vi "main_grid_forming_PQ_bu.vi"() -> ()   [LabVIEW 2021]
uses:
  <vilib>/xnet/xnet.llb/XNET Frame CAN.ctl
  <vilib>/xnet/xnet.llb/XNET Frame Type CAN.ctl
  Helper functions/General Purpose/references.ctl
  Helper functions/General Purpose/measurements.ctl
  Helper functions/Time-sync/time_sync/TypeDef/Synch_shift--cluster.ctl
  <vilib>/Platform/TimedLoop/XDataNode/timing_clust.ctl
  <vilib>/Platform/TimedLoop/XDataNode/nitl_modes.ctl
  <vilib>/Platform/TimedLoop/XDataNode/wakeup.ctl
  Helper functions/communication/AFE_froming_Central.ctl
  Helper functions/communication/AFE_froming_Central_Info.ctl
  Helper functions/communication/AFE_froming_Central_Data.ctl
  <vilib>/xnet/xnet.llb/XNET Write (Frame CAN).vi
  <vilib>/xnet/xnet.llb/XNET Read (Frame CAN).vi
  <vilib>/Platform/TimedLoop/XDataNode/XDataNode.xnode
  <vilib>/Platform/TimedLoop/XDataNode/XDNodeRunTimeDep.lvlib
  <userlib>/_OpenG.lib/boolean/boolean.llb/openg_boolean__ogtk.lvlib
panel:
  in  "Q2 bias":dbl=-800.0
  in  "delta V":dbl format="%#_13g"
  in  "delta f":dbl=0.005800000000000027 format="%#_13g"
  in  "biasQ4":dbl=200.0
  in  "biasV4":dbl
  in  "biasV1":dbl=0.6
  out "form":timestamp
  out "follow":timestamp
  out "time_afe":timestamp
  out "start following 1 pre":bool
  out "t_rising":timestamp
  out "t_risingedge":dbl
  out "Synch Monitor":string[][](table)
  in  "Loop Time":u32=125
  out "Error out":errorcluster
  in  "Timeout [ms]":i32=3000
  out "Offset from TR (ns)":dbl
  out "Status Out":T1
  out "CAN OUT":T2[](array[typedef]) {"payload" format="%x"; "timestamp" format="%<%.7X\n%x>T"; "type" items=["CAN Data"=0, "CAN Remote"=1, "CAN Bus Error"=2, "CAN 2.0 Data"=8, "CAN FD Data"=16, "CAN FD+BRS Data"=24, "J1939 Data"=192, "Delay"=224, "Log Trigger"=225, "Start Trigger"=226]; "identifier" format="%x"}
  in  "freq 1":dbl=50.0
  in  "Vabs 1":dbl=230.0
  in  "Varg 1":dbl
  in  "Start following 1":bool
  out "Forming 2":bool
  out "Forming 1":bool
  in  "Start forming 1":bool
  out "current time":timestamp
  in  "measurements":T4
  in  "references":T5
  in  "To ACT CH 4":bool
  in  "To ACT CH 3":bool
  in  "To ACT CH 2":bool
  out "Error 4":bool
  out "Fault 4":bool
  out "Error 3":bool
  out "Fault 3":bool
  out "Error 2":bool
  out "Fault 2":bool
  out "State code 4":i32
  out "State code 3":i32
  out "State code 2":i32
  out "State code 1":i32
  out "Error 1":bool
  out "Fault 1":bool
  in  "To ACT CH 1":bool
  in  "main stop":bool
  in  "Vdc4":dbl=750.0
  in  "Qac4":dbl
  in  "Pac3":dbl=750.0
  in  "Qac3":dbl
  in  "Pac2":dbl
  in  "Qac2":dbl
  in  "Emergency 4":bool
  in  "To IN OP  4":bool
  in  "SEND sp 4":bool
  in  "Clear 4":bool
  in  "Shutdwn 4":bool
  in  "Emergency 3":bool
  in  "To IN OP  3":bool
  in  "SEND sp 3":bool
  in  "Clear 3":bool
  in  "Shutdwn 3":bool
  in  "Emergency 2":bool
  in  "To IN OP  2":bool
  in  "SEND sp 2":bool
  in  "Clear 2":bool
  in  "Shutdwn 2":bool
  out "V slider 22":dbl(slide) caption="V-i" max=-10.0 scale=650.0..780.0 scale format="%#_4g"
  out "V slider 21":dbl(slide) caption="V-i" max=-10.0 scale=650.0..780.0 scale format="%#_4g"
  out "V slider 20":dbl(slide) caption="V-i" max=-10.0 scale=650.0..780.0 scale format="%#_4g"
  out "kW":dbl caption="Numeric" format="%#.3g"
  out "?VkVAr":dbl caption="Numeric" format="%.3g"
  out "kW":dbl caption="Numeric" format="%#.3g"
  out "?VkVAr":dbl caption="Numeric" format="%.3g"
  out "kW":dbl caption="Numeric" format="%#.3g"
  out "?VkVAr":dbl caption="Numeric" format="%.3g"
  out "OFF 4":bool
  out "ON 4":bool
  out "Ready 4":bool
  out "OFF 3":bool
  out "ON 3":bool
  out "Ready 3":bool
  out "OFF 2":bool
  out "ON 2":bool
  out "Ready 2":bool
  out "error out":errorcluster
  out "?VkVAr":dbl caption="Numeric" format="%.3g"
  out "kW":dbl caption="Numeric" format="%#.3g"
  out "V slider 19":dbl(slide) caption="V-i" max=-10.0 scale=650.0..780.0 scale format="%#_4g"
  in  "Vdc1":dbl=750.0
  out "OFF 1":bool
  out "ON 1":bool
  out "Ready 1":bool
  out "CAN IN":T2 {"payload" format="%x"; "timestamp" format="%<%.7X\n%x>T"; "type" items=["CAN Data"=0, "CAN Remote"=1, "CAN Bus Error"=2, "CAN 2.0 Data"=8, "CAN FD Data"=16, "CAN FD+BRS Data"=24, "J1939 Data"=192, "Delay"=224, "Log Trigger"=225, "Start Trigger"=226]; "identifier" format="%x"}
  in  "Emergency 1":bool
  in  "Qac1":dbl
  in  "conv":T6
  in  "CAN [ms]":i64=1
  out "CAN with Conv":bool
  out "Measurements":bool
  in  "Shutdwn 1":bool
  in  "Clear 1":bool
  in  "SEND sp 1":bool
  in  "To IN OP 1":bool
  out "logging":bool
  # "Resource agents: AFE 1-4"
  # "package identifiers:\n1xx VSC1 \n2xx VSC2\n3xx VSC3\n4xx VSC4\n\nx0x send from agent to resource\nx02 Power setpoints\nx06 Measurements\nx9 status\n          = [state; error; alarm; OFF; Ready; ON]\n\n \n\nx1x send from resource to agent\nx10 Power measurements\nx11 Measurements\nx12 status\n          = [state; error; alarm; full; precharge; neg; 0; 0]"
  # "B18"
  # "B 22\nB19"
  # "VSC 4"
  # "B17"
  # "B21"
  # "VSC 3"
  # "B16"
  # "B20"
  # "Start-up - Shut down"
  # "VSC 2"
  # "B15"
  # "B19"
  # "Start-up - Shut down"
  # "VSC 1"
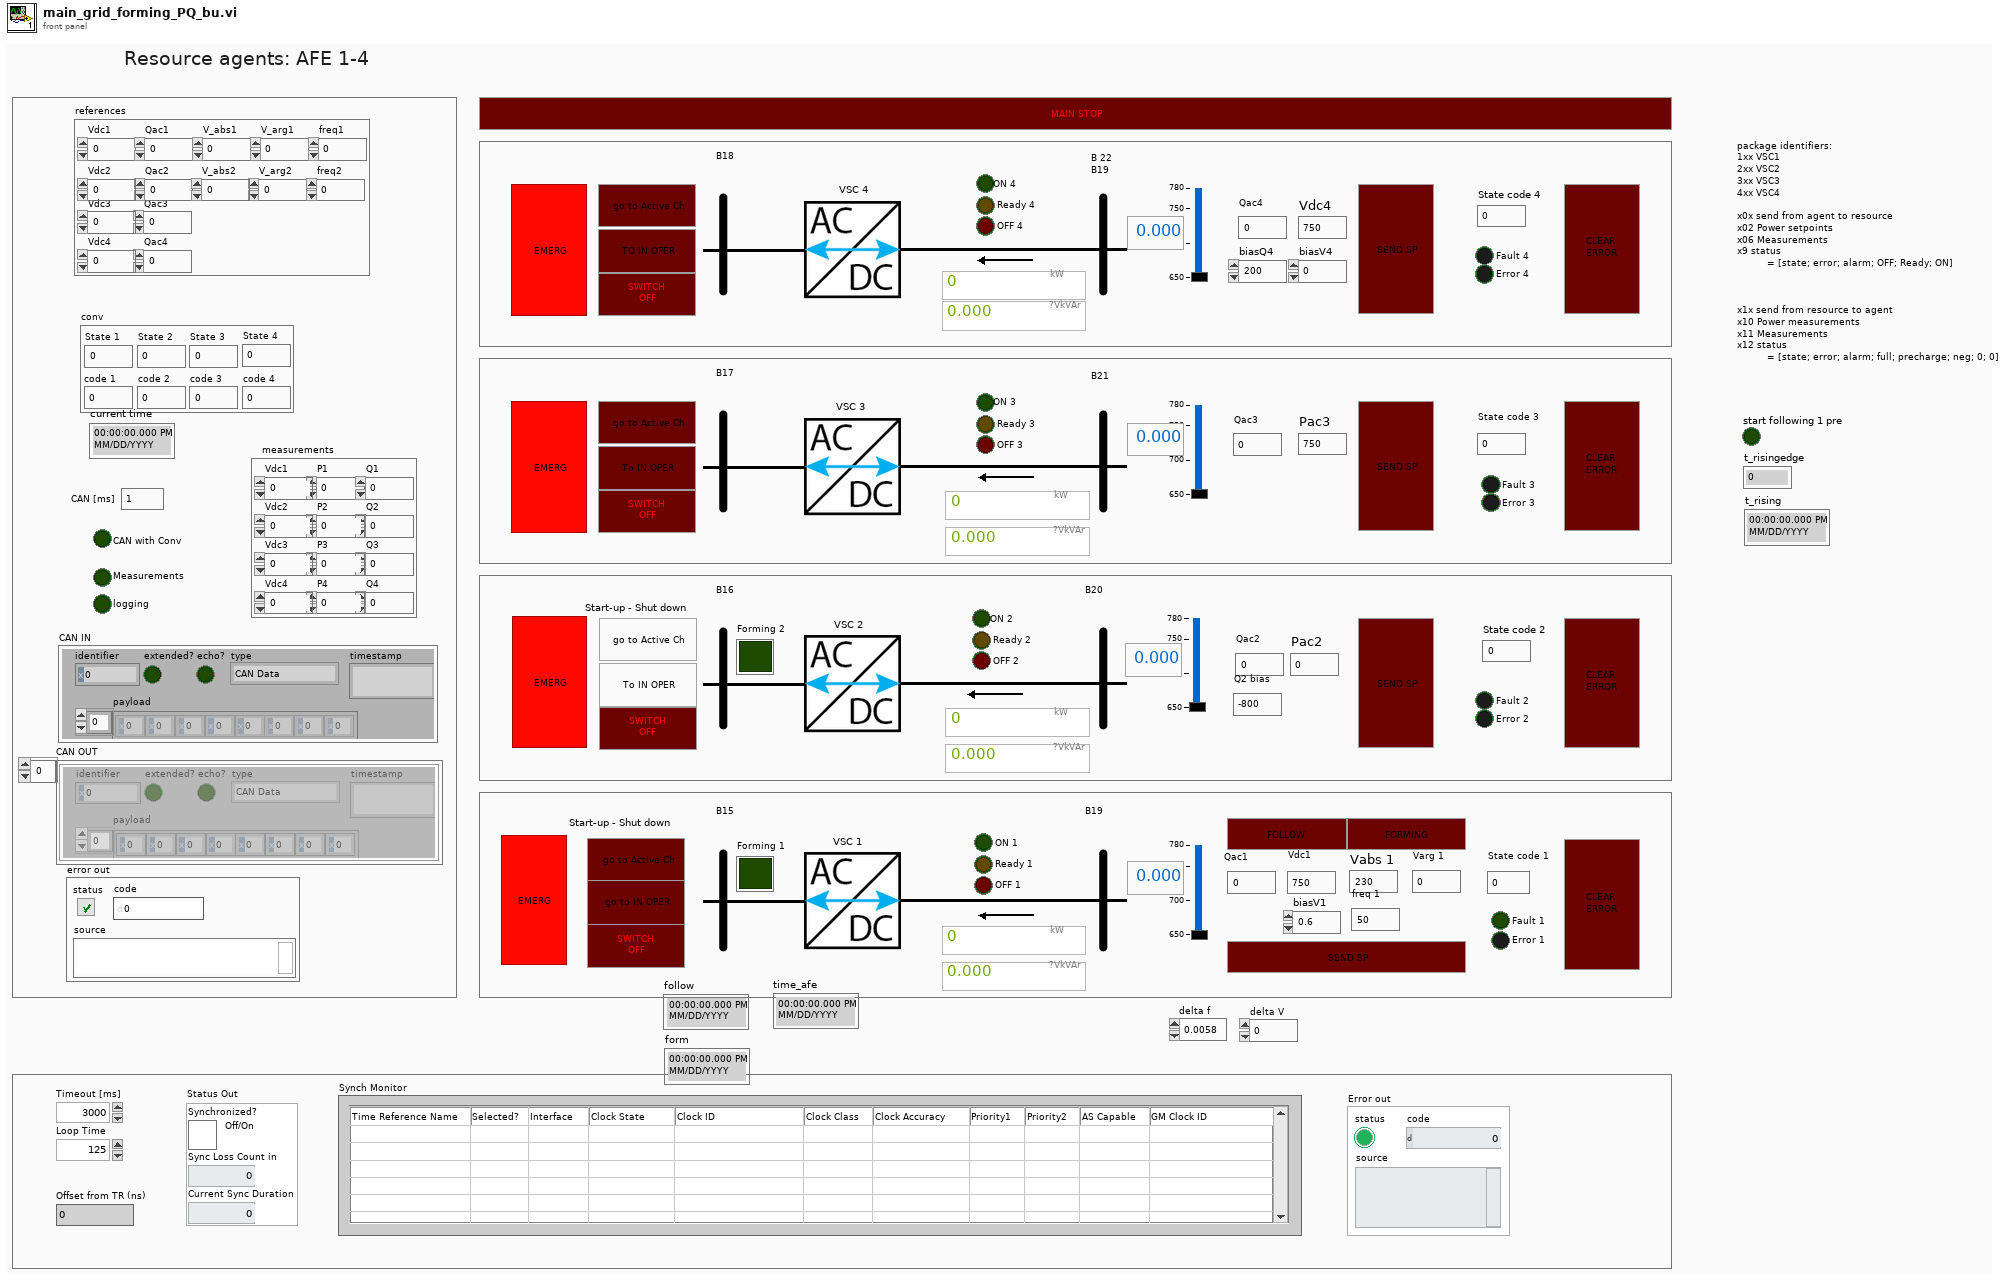
[diagram p1: front panel]
types:
  T1 = typedef "Synch_shift--cluster.ctl" = cluster{"Synchronized?":bool, "Sync Loss Count in":u32, "Current Sync Duration":u32}
  T2 = typedef "XNET Frame CAN.ctl" = cluster{"timestamp":timestamp, "payload":u8[], "identifier":u32, "type":T3, "extended?":bool, "echo?":bool}
  T3 = typedef "XNET Frame Type CAN.ctl" = u8
  T4 = typedef "measurements.ctl" = cluster{"Vdc1":dbl, "P1":dbl, "Vdc2":dbl, "P2":dbl, "Q2":dbl, "Vdc3":dbl, "P3":dbl, "Q3":dbl, "Vdc4":dbl, "P4":dbl, "Q4":dbl, "Q1":dbl}
  T5 = typedef "references.ctl" = cluster{"Vdc1":dbl, "Vdc2":dbl, "Qac2":dbl, "Vdc3":dbl, "Qac3":dbl, "Vdc4":dbl, "Qac4":dbl, "Qac1":dbl, "V_arg2":dbl, "V_abs2":dbl, "V_abs1":dbl, "V_arg1":dbl, "freq1":dbl, "freq2":dbl}
  T6 = cluster{"State 1":dbl, "code 1":dbl, "code 2":dbl, "code 3":dbl, "code 4":dbl, "State 2":dbl, "State 3":dbl, "State 4":dbl}
  T7 = cluster{"Frame In":refnum<k21>, "Frame Out":refnum<k21>}
  T8 = typedef "XDNodeRunTimeDep.lvlib/timing_clust.ctl" = cluster{"Expected End [f-1]":u64, "Actual End [f-1]":u64, "Finished Late? [f-1]":bool, "Expected End [i-1]":u64, "Actual End [i-1]":u64, "Finished Late? [i-1]":bool, "Expected Start [i]":u64, "Actual Start [i]":u64, "Expected Start [f]":u64, "Actual Start [f]":u64, "Source Name":string, "Structure Name":string, "Period":i64, "Deadline":i64, "Offset":i64, "Start":i64, "Priority":i32, "Timeout":i32, "Mode":T9, "Wakeup Reason":T10, "Error":errorcluster, "Source Type":string, "Secondary Source Type":string, "Global End Time":u64, "Global Start Time":u64, "Frame Duration":u64, "Iteration Duration":u64, "Assigned CPU":i32, "I/O Scan Engine Mode":u32}
  T9 = typedef "XDNodeRunTimeDep.lvlib/nitl_modes.ctl" = enum32{"No Change", "Process missed periods, maintain original phase", "Discard missed periods, maintain original phase", "Process missed periods, ignore original phase", "Discard missed periods, ignore original phase"}
  T10 = typedef "XDNodeRunTimeDep.lvlib/wakeup.ctl" = enum32{"Normal", "Aborted", "Asynchronous wakeup", "Timing source error", "Timed loop error", "Timeout"}
  T11 = typedef "AFE_froming_Central.ctl" = cluster{"Info":T12, "Data":T13}
  T12 = typedef "AFE_froming_Central_Info.ctl" = cluster{"Resource":string, "Problem":bool, "Timestamp":dbl}
  T13 = typedef "AFE_froming_Central_Data.ctl" = cluster{"Start forming 1":bool, "Forming/Following":bool[], "Start forming 2":bool, "measurements":cluster{"Vdc1":dbl, "P1":dbl, "Vdc2":dbl, "P2":dbl, "Q2":dbl, "Vdc3":dbl, "P3":dbl, "Q3":dbl, "Vdc4":dbl, "P4":dbl, "Q4":dbl, "Q1":dbl}, "Status":bool[], "references":T5, "Start following 1":bool, "Start following 2":bool}
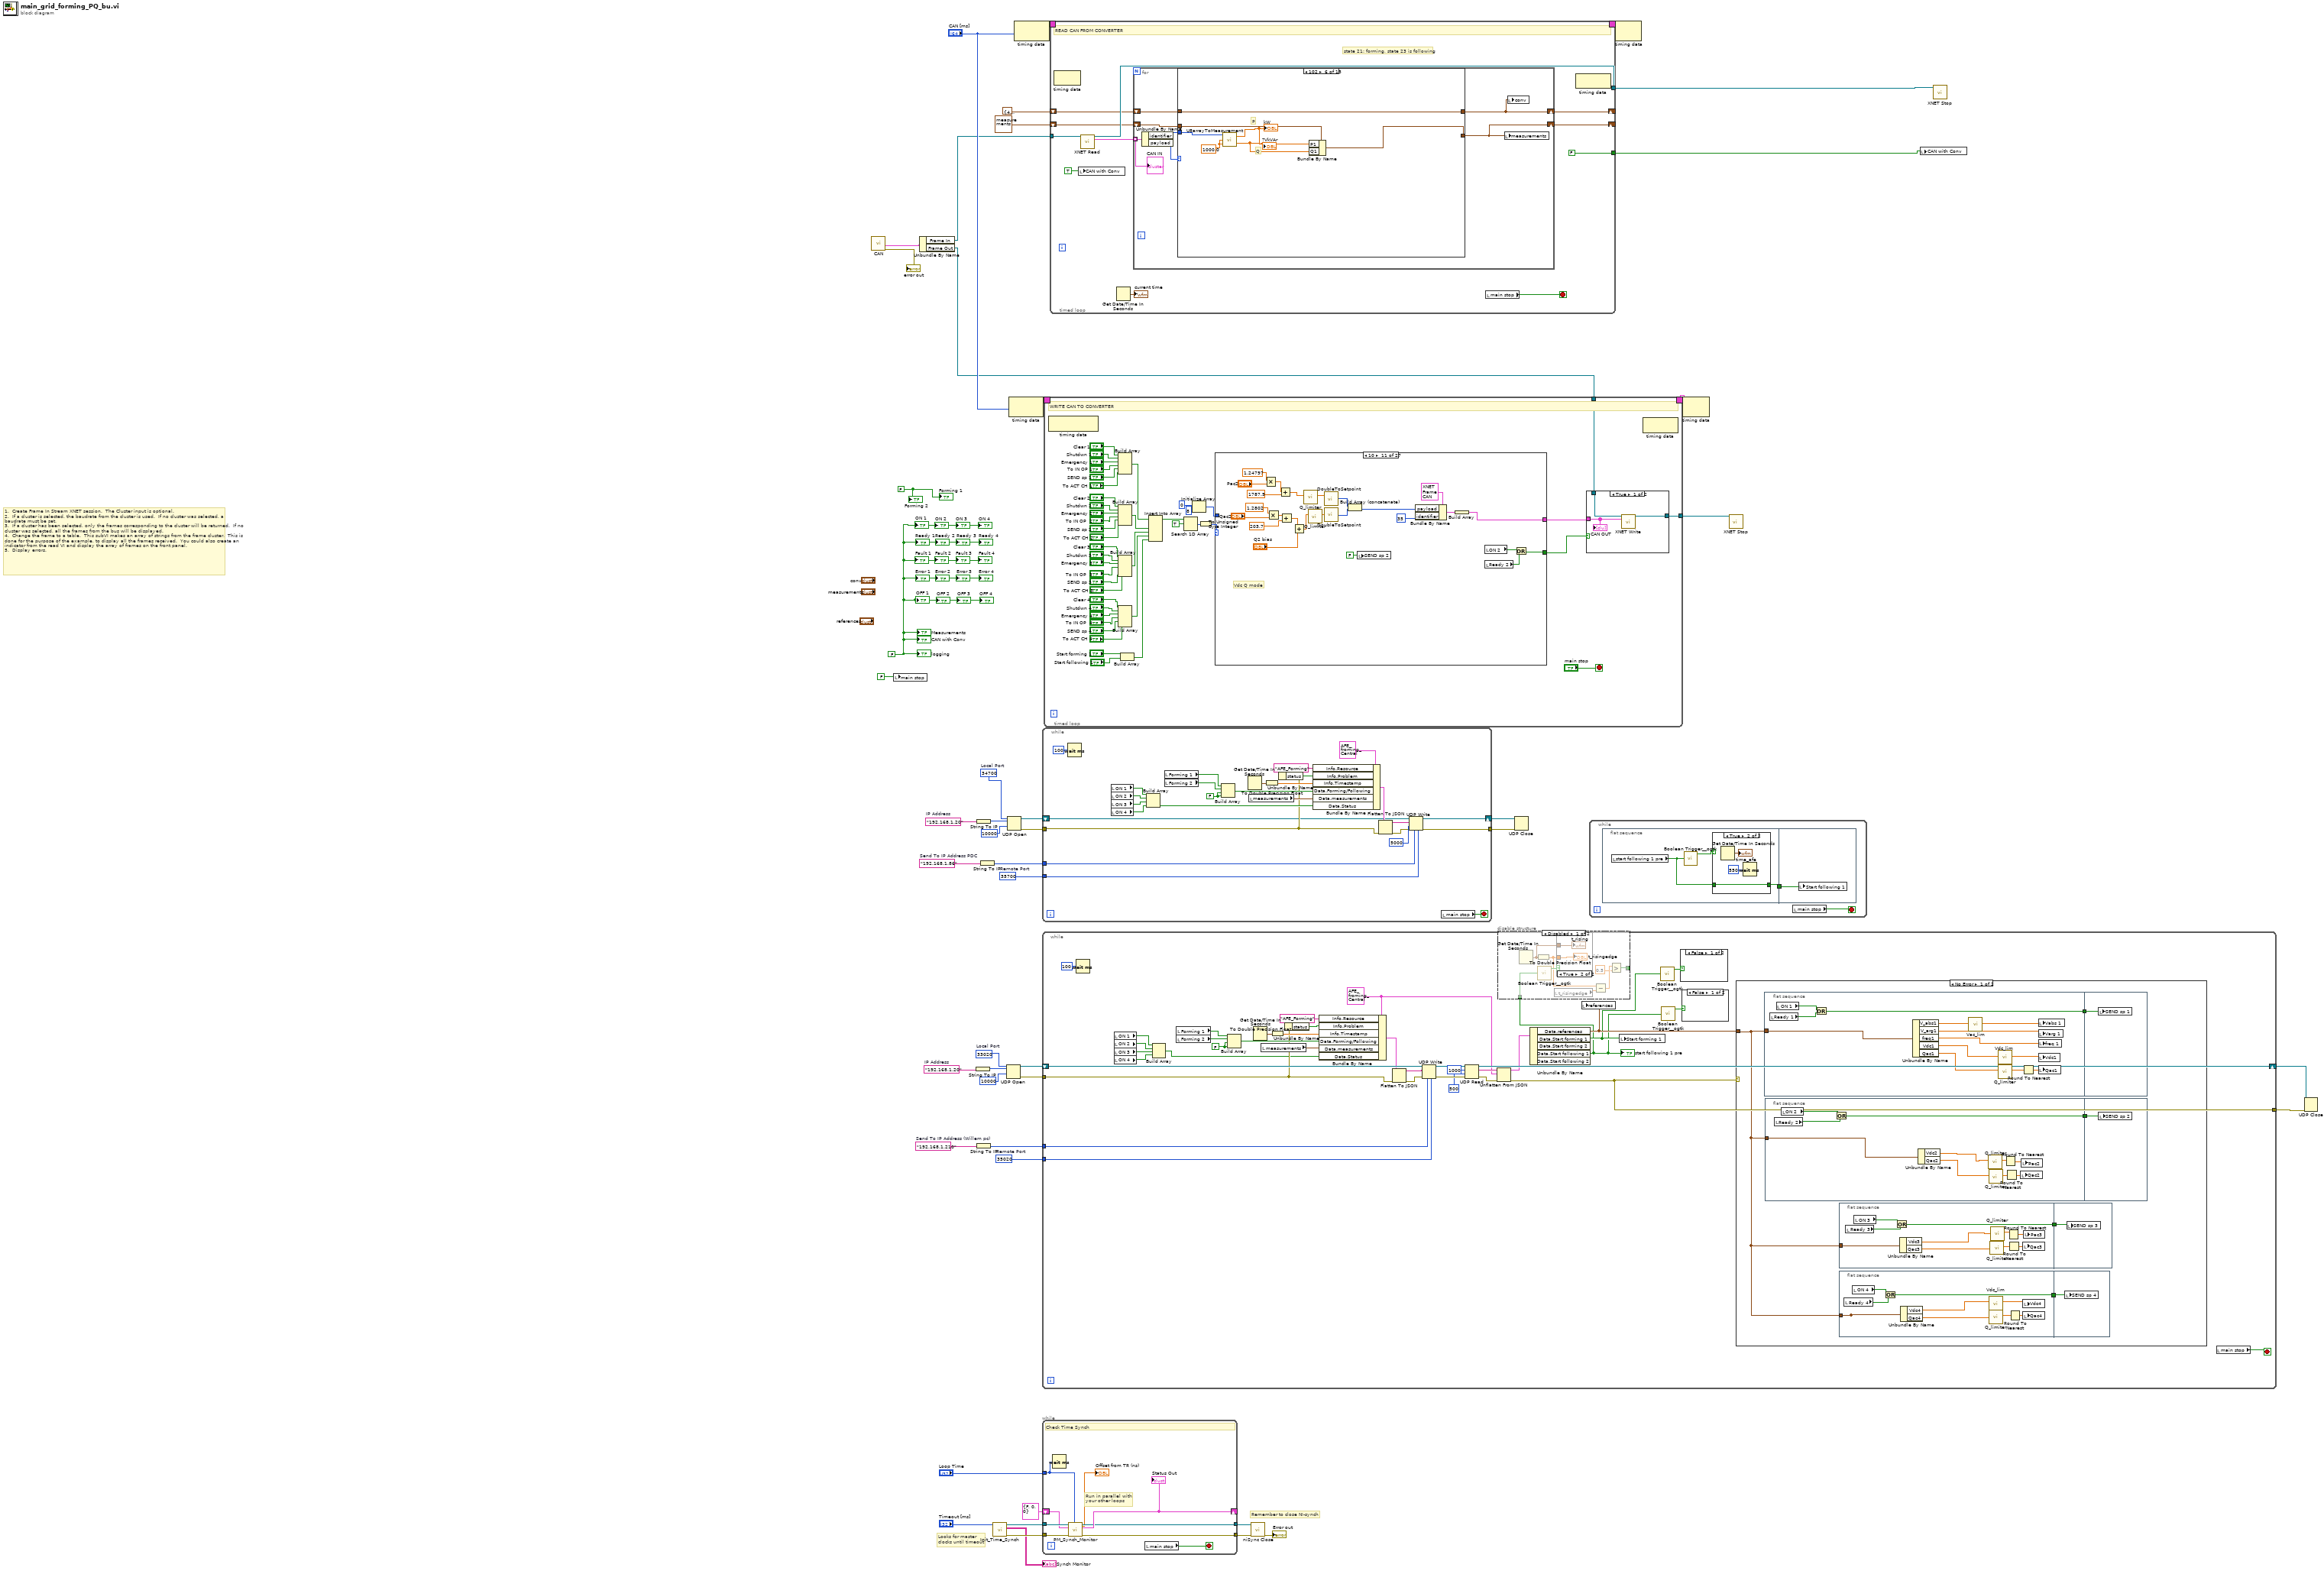
[diagram p0: block diagram]
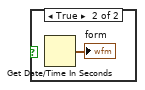
[diagram p3: hidden frame]
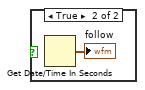
[diagram p4: hidden frame]
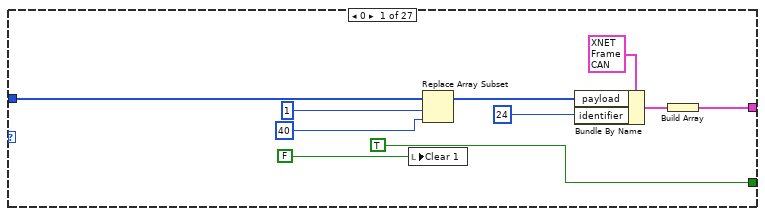
[diagram p9: hidden frame]
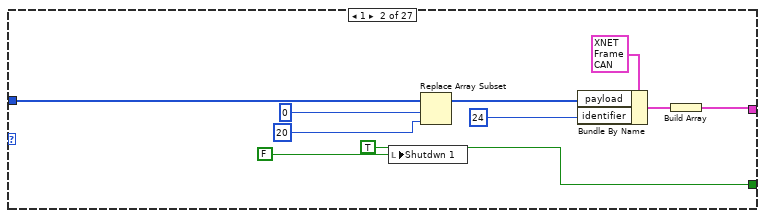
[diagram p10: hidden frame]
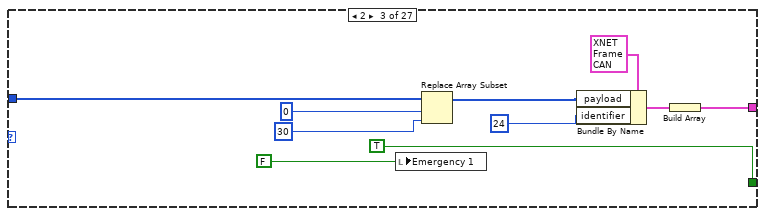
[diagram p11: hidden frame]
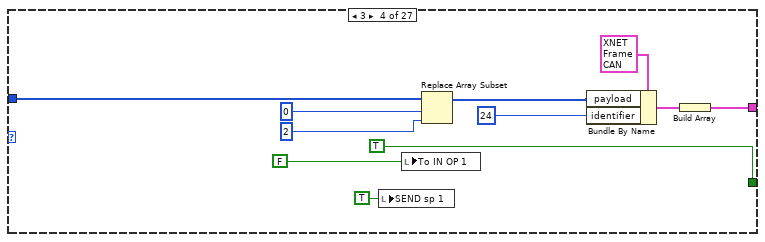
[diagram p12: hidden frame]
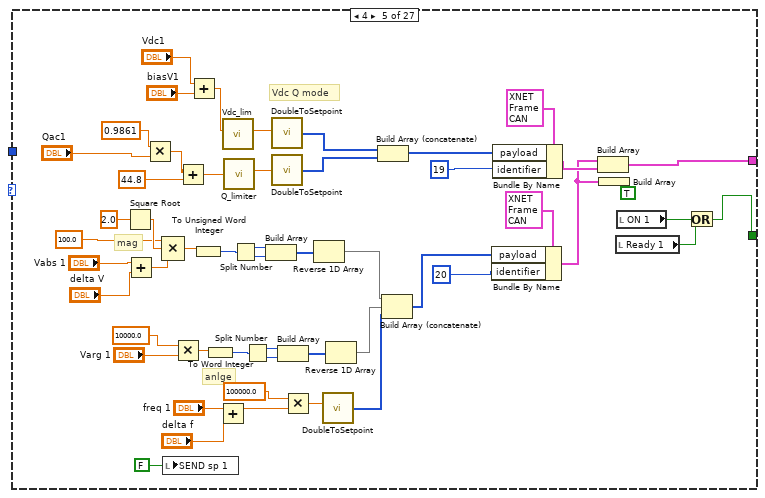
[diagram p13: hidden frame]
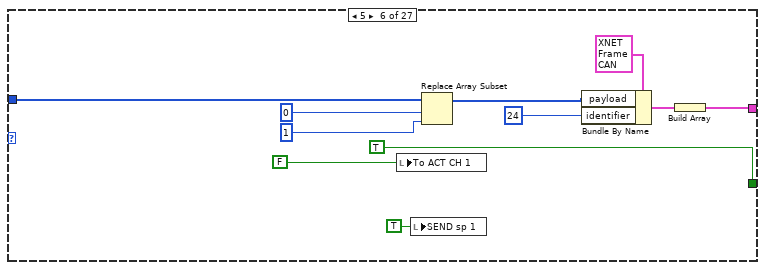
[diagram p14: hidden frame]
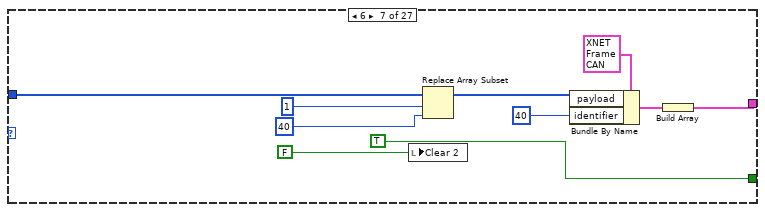
[diagram p15: hidden frame]
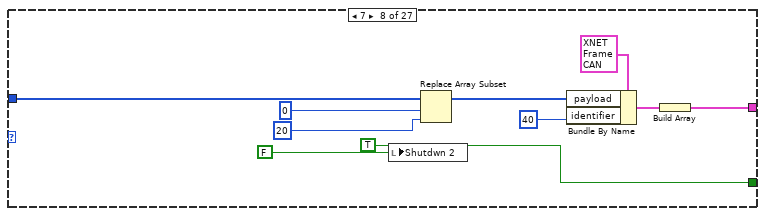
[diagram p16: hidden frame]
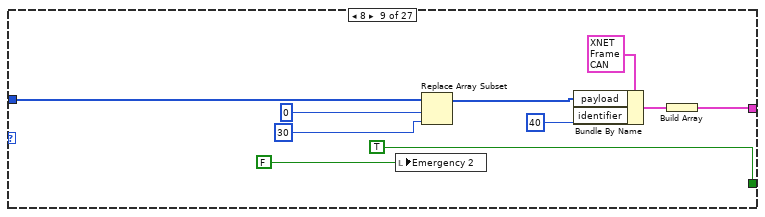
[diagram p17: hidden frame]
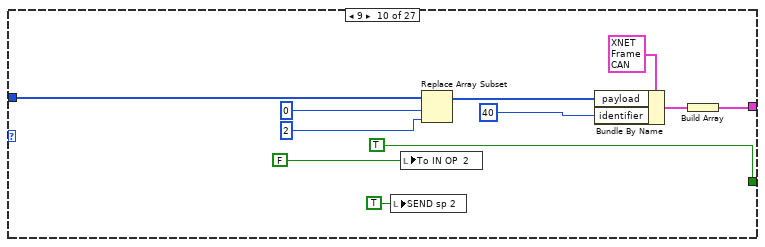
[diagram p18: hidden frame]
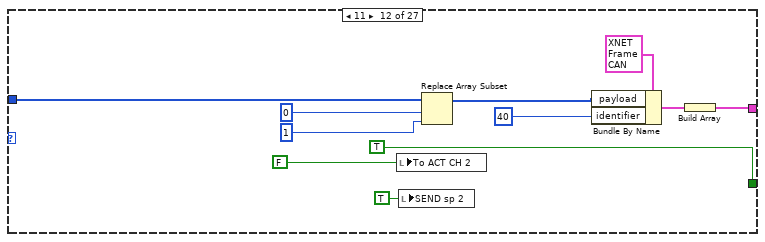
[diagram p19: hidden frame]
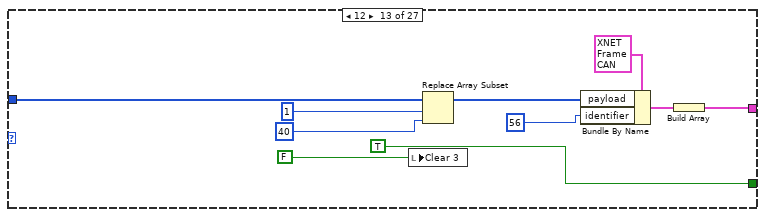
[diagram p20: hidden frame]
diagram:
  w7 = u16 35020  # Remote Port
  w13 = "192.168.1.210"  # Send To IP Address (Willem pc)
  w15 = u16 33020  # Local Port
  w16 = "192.168.1.20"  # IP Address
  w28 = FALSE ("Forming")
  w4 = u16 35700  # Remote Port
  w29 = "192.168.1.86"  # Send To IP Address PDC
  w31 = u16 34700  # Local Port
  w32 = "192.168.1.20"  # IP Address
  w34 = FALSE
  # "Remember to close NI-synch"
  # "Looks for master \nclocks until timeout"
  # "1.  Create Frame In Stream XNET session.  The Cluster input is optional.  \n2.  If a cluster is selected, the baudrate from the cluster is used.  If no cluster was selected, a baudrate must be set.\n3.  If a cluster has been selected, only the frames corresponding to the cluster will be returned.  If no cluster was selected, all the frames from the bus will be displayed.\n4.  Change the frame to a table.  This subVI makes an array of strings from the frame cluster.  This is done for the purpose of the example, to display all the frames received.  You could also create an indicator from the read VI and display the array of frames on the front panel. \n5.  Display errors."
  n1 = call "CAN.vi"() -> ("error out"=→"error out":errorcluster, "CAN"=w36:T7)  [unwired: 10 in]
  n2 = local write "main stop"(FALSE ("main stop")) -> ()
  n3 = Unbundle By Name(w36) -> ("Frame In"=w41:refnum<k21>, "Frame Out"=w44:refnum<k21>)
  n4 = String To IP(1:w16) -> (0:w17:u32)
  n5 = String To IP(1:w32) -> (0:w33:u32)
  n6 = String To IP(1:w13) -> (0:w8:u32)
  n7 = String To IP(1:w29) -> (0:w5:u32)
  n8 = call "Init_Time_Synch.vi"("Timeout [ms]"="Timeout [ms]") -> ("Error out"=w25:errorcluster, "Synch Monitor"=→"Synch Monitor":string[][], "Synch Out"=w23:refnum<k15>)  [unwired: 7 in, 1 out]
  n9 = UDP Open(7:w17, 9:10000 ("timeout ms (25000)"), 11:w15) -> (port=w12:refnum<k16>, 0:w11:errorcluster)  [unwired: 2 in, 1 out]
  n10 = UDP Open(7:w33, 9:10000 ("timeout ms (25000)"), 11:w31) -> (port=w3:refnum<k16>, 0:w2:errorcluster)  [unwired: 2 in, 1 out]
  n11 = node-c288("CAN [ms]") -> (w38:T8)
  n12 = node-c288("CAN [ms]") -> (w43:T8)
  n13 = while {
    tunnel: w11 -> [w64]
    shift-right: [w81] -> w10
    shift-left: w12 -> [w83]
    tunnel: [w84] -> w9
    tunnel: w8 -> [w73]
    tunnel: w7 -> [w77]
    stop <- w86 stop-if-true
    w61 = FALSE ("ON 1")
    w54 = T11 {"Info"={"Resource"="AFE_Forming", "Problem"=FALSE, "Timestamp"=0.0}, "Data"={"Start forming 1"=FALSE, "Forming/Following"=[], "Start forming 2"=FALSE, "measurements"={"Vdc1"=0.0, "P1"=0.0, "Vdc2"=0.0, "P2"=0.0, "Q2"=0.0, "Vdc3"=0.0, "P3"=0.0, "Q3"=0.0, "Vdc4"=0.0, "P4"=0.0, "Q4"=0.0, "Q1"=0.0}, "Status"=[], "references"={"Vdc1"=0.0, "Vdc2"=0.0, "Qac2"=0.0, "Vdc3"=0.0, "Qac3"=0.0, "Vdc4"=0.0, "Qac4"=0.0, "Qac1"=0.0, "V_arg2"=0.0, "V_abs2"=0.0, "V_abs1"=0.0, "V_arg1"=0.0, "freq1"=0.0, "freq2"=0.0}, "Start following 1"=FALSE, "Start following 2"=FALSE}} ("Cluster")
    n14 = Wait (ms)(milliseconds to wait=u32 100) -> ()  [unwired: 1 out]
    n15 = local read "ON 1"() -> (w59:bool)
    n16 = local read "ON 2"() -> (w60:bool)
    n17 = local read "ON 3"() -> (w57:bool)
    n18 = local read "ON 4"() -> (w56:bool)
    n19 = Build Array(w59, w60, w57, w56) -> (w58:bool[])
    n20 = local read "Forming 1"() -> (w63:bool)
    n21 = local read "Forming 2"() -> (w62:bool)
    n22 = Build Array(w63, w62, w61, w61) -> (w70:bool[])
    n23 = Get Date/Time In Seconds() -> (seconds since 1Jan1904=w66:timestamp)
    n24 = local read "measurements"() -> (w55:T4)
    n25 = To Double Precision Float(number=w66) -> (double precision float=w69:dbl)
    n26 = Unbundle By Name(w64) -> ("status"=w65:bool)
    n27 = Bundle By Name(cluster=w54, "Info.Resource"="AFE_Forming", "Info.Problem"=w65, "Info.Timestamp"=w69, "Data.Forming/Following"=w70, "Data.measurements"=w55, "Data.Status"=w58) -> (w67:T11)
    n28 = Flatten To JSON(anything=w67, error in (no error)=w64) -> (JSON string=w72:string, 11:w71:errorcluster)  [unwired: 1 in]
    n29 = UDP Write(address=w73, port or service name=w77, connection ID=w83, data in=w72, 8:w71) -> (error out=w79:errorcluster, 3:w82:refnum<k16>)  [unwired: 1 in]
    n30 = UDP Read(connection ID=w82, max size (548)=1000, timeout ms (25000)=500, 8:w79) -> (data out=w80:string, error out=w76:errorcluster, 3:w81:refnum<k16>)  [unwired: 2 out]
    n31 = Unflatten From JSON(JSON string=w80, type and defaults=w54, error in (no error)=w76) -> (value=w74:T11, error out=w84:errorcluster)  [unwired: 4 in]
    n32 = Unbundle By Name(w74) -> ("Data.references"=w85:T5, "Data.Start forming 1"=w50:bool, "Data.Start following 1"=w49:bool)  [unwired: 2 out]
    "start following 1 pre" <- w49
    n33 = disable-structure shown="Disabled" {
      disable-tunnel: [w93 _] -> _
      disable-tunnel: w49 -> [w91 _]
      frame Disabled {
        n34 = Get Date/Time In Seconds() -> (seconds since 1Jan1904=w92:timestamp)
        n35 = To Double Precision Float(number=w92) -> (double precision float=w94:dbl)
        n36 = call <userlib>:"Boolean Trigger__ogtk.vi"("Boolean Input"=w91) -> ("Rising Edge"=w96:bool)  [unwired: 1 in, 1 out]
        n37 = local read "t_risingedge"() -> (w95:dbl)
        n38 = case shown="True" w96 {
          tunnel: w94 -> [_ w98]
          tunnel: w92 -> [_ w97]
          frame False {
          }
          frame True {
            "t_risingedge" <- w98
            "t_rising" <- w97
          }
        }
        n39 = Subtract(x=w94, y=w95) -> (x-y=w90:dbl)
        n40 = Greater?(x=w90, y=0.5 ("x")) -> (0:w93:bool)
      }
      frame Enabled {
      }
    }
    n41 = local write "references"(w85) -> ()
    n42 = local write "Start forming 1"(w50) -> ()
    n43 = call <userlib>:"Boolean Trigger__ogtk.vi"("Boolean Input"=w50) -> ("Rising Edge"=w51:bool)  [unwired: 1 in, 1 out]
    n44 = call <userlib>:"Boolean Trigger__ogtk.vi"("Boolean Input"=w49) -> ("Rising Edge"=w52:bool)  [unwired: 1 in, 1 out]
    n45 = case shown="False" w51 {
      frame False {
      }
      frame True {
        n46 = Get Date/Time In Seconds() -> (seconds since 1Jan1904=→"form":timestamp)
      }
    }
    n47 = case shown="False" w52 {
      frame False {
      }
      frame True {
        n48 = Get Date/Time In Seconds() -> (seconds since 1Jan1904=→"follow":timestamp)
      }
    }
    n49 = case shown="No Error" w84 {
      tunnel: w85 -> [w103 _]
      frame No Error {
        n50 = flat-sequence {
          tunnel: w103 -> [w148]
          tunnel: [w138] -> w101
          tunnel: w101 -> [w149]
          frame #0 {
            n51 = local read "Ready 1"() -> (w140:bool)
            n52 = local read "ON 1"() -> (w139:bool)
            n53 = Or(x=w139, y=w140) -> (x .or. y?=w138:bool)
            n54 = Unbundle By Name(w148) -> ("V_abs1"=w146:dbl, "V_arg1"=w147:dbl, "freq1"=w144:dbl, "Vdc1"=w136:dbl, "Qac1"=w141:dbl)
            n55 = call "Vac_lim.vi"("IN Vdc"=w146) -> ("OUT Vdc"=w145:dbl)  [unwired: 10 in]
            n56 = call "Vdc_lim.vi"("IN Vdc"=w136) -> ("OUT Vdc"=w143:dbl)  [unwired: 10 in]
            n57 = call "Q_limiter.vi"("IN Q"=w141) -> ("OUT Q"=w142:dbl)  [unwired: 10 in]
            n58 = Round To Nearest(number=w142) -> (nearest integer value=w137:dbl)
            n59 = local write "Vabs 1"(w145) -> ()
            n60 = local write "Varg 1"(w147) -> ()
            n61 = local write "freq 1"(w144) -> ()
            n62 = local write "Vdc1"(w143) -> ()
            n63 = local write "Qac1"(w137) -> ()
          }
          frame #1 {
            n64 = local write "SEND sp 1"(w149) -> ()
          }
        }
        n65 = flat-sequence {
          tunnel: w103 -> [w134]
          tunnel: [w129] -> w102
          tunnel: w102 -> [w135]
          frame #0 {
            n66 = local read "Ready 2"() -> (w131:bool)
            n67 = local read "ON 2"() -> (w130:bool)
            n68 = Or(x=w130, y=w131) -> (x .or. y?=w129:bool)
            n69 = Unbundle By Name(w134) -> ("Vdc2"=w125:dbl, "Qac2"=w132:dbl)
            n70 = call "Q_limiter.vi"("IN Q"=w125) -> ("OUT Q"=w126:dbl)  [unwired: 10 in]
            n71 = call "Q_limiter.vi"("IN Q"=w132) -> ("OUT Q"=w133:dbl)  [unwired: 10 in]
            n72 = Round To Nearest(number=w126) -> (nearest integer value=w127:dbl)
            n73 = Round To Nearest(number=w133) -> (nearest integer value=w128:dbl)
            n74 = local write "Qac2"(w128) -> ()
            n75 = local write "Pac2"(w127) -> ()
          }
          frame #1 {
            n76 = local write "SEND sp 2"(w135) -> ()
          }
        }
        n77 = flat-sequence {
          tunnel: w103 -> [w123]
          tunnel: [w120] -> w100
          tunnel: w100 -> [w124]
          frame #0 {
            n78 = local read "Ready 3"() -> (w121:bool)
            n79 = local read "ON 3"() -> (w119:bool)
            n80 = Or(x=w119, y=w121) -> (x .or. y?=w120:bool)
            n81 = Unbundle By Name(w123) -> ("Vdc3"=w116:dbl, "Qac3"=w122:dbl)
            n82 = call "Q_limiter.vi"("IN Q"=w122) -> ("OUT Q"=w118:dbl)  [unwired: 10 in]
            n83 = call "Q_limiter.vi"("IN Q"=w116) -> ("OUT Q"=w115:dbl)  [unwired: 10 in]
            n84 = Round To Nearest(number=w115) -> (nearest integer value=w114:dbl)
            n85 = Round To Nearest(number=w118) -> (nearest integer value=w117:dbl)
            n86 = local write "Qac3"(w117) -> ()
            n87 = local write "Pac3"(w114) -> ()
          }
          frame #1 {
            n88 = local write "SEND sp 3"(w124) -> ()
          }
        }
        n89 = flat-sequence {
          tunnel: [w112] -> _
          tunnel: w103 -> [w112]
          tunnel: [w106] -> w99
          tunnel: w99 -> [w113]
          frame #0 {
            n90 = local read "Ready 4"() -> (w108:bool)
            n91 = local read "ON 4"() -> (w107:bool)
            n92 = Or(x=w107, y=w108) -> (x .or. y?=w106:bool)
            n93 = Unbundle By Name(w112) -> ("Vdc4"=w104:dbl, "Qac4"=w109:dbl)
            n94 = call "Vdc_lim.vi"("IN Vdc"=w104) -> ("OUT Vdc"=w111:dbl)  [unwired: 10 in]
            n95 = call "Q_limiter.vi"("IN Q"=w109) -> ("OUT Q"=w110:dbl)  [unwired: 10 in]
            n96 = Round To Nearest(number=w110) -> (nearest integer value=w105:dbl)
            n97 = local write "Vdc4"(w111) -> ()
            n98 = local write "Qac4"(w105) -> ()
          }
          frame #1 {
            n99 = local write "SEND sp 4"(w113) -> ()
          }
        }
      }
      frame Error {
      }
    }
    n100 = local read "main stop"() -> (w86:bool)
  }
  n101 = while {
    tunnel: [w156] -> w6
    tunnel: w5 -> [w154]
    tunnel: w4 -> [w155]
    tunnel: w2 -> [w153]
    shift-right: [w151] -> w1
    shift-left: w3 -> [w152]
    stop <- w150 stop-if-true
    w173 = FALSE ("ON 1")
    n102 = Wait (ms)(milliseconds to wait=u32 100) -> ()  [unwired: 1 out]
    n103 = local read "ON 1"() -> (w166:bool)
    n104 = local read "ON 2"() -> (w165:bool)
    n105 = local read "ON 3"() -> (w167:bool)
    n106 = local read "ON 4"() -> (w168:bool)
    n107 = Build Array(w166, w165, w167, w168) -> (w169:bool[])
    n108 = local read "Forming 1"() -> (w172:bool)
    n109 = local read "Forming 2"() -> (w171:bool)
    n110 = Build Array(w172, w171, w173, w173) -> (w170:bool[])
    n111 = Get Date/Time In Seconds() -> (seconds since 1Jan1904=w161:timestamp)
    n112 = local read "measurements"() -> (w164:T4)
    n113 = To Double Precision Float(number=w161) -> (double precision float=w162:dbl)
    n114 = Unbundle By Name(w153) -> ("status"=w174:bool)
    n115 = Bundle By Name(cluster=T11 {"Info"={"Resource"="AFE_Forming", "Problem"=FALSE, "Timestamp"=0.0}, "Data"={"Start forming 1"=FALSE, "Forming/Following"=[], "Start forming 2"=FALSE, "measurements"={"Vdc1"=0.0, "P1"=0.0, "Vdc2"=0.0, "P2"=0.0, "Q2"=0.0, "Vdc3"=0.0, "P3"=0.0, "Q3"=0.0, "Vdc4"=0.0, "P4"=0.0, "Q4"=0.0, "Q1"=0.0}, "Status"=[], "references"={"Vdc1"=0.0, "Vdc2"=0.0, "Qac2"=0.0, "Vdc3"=0.0, "Qac3"=0.0, "Vdc4"=0.0, "Qac4"=0.0, "Qac1"=0.0, "V_arg2"=0.0, "V_abs2"=0.0, "V_abs1"=0.0, "V_arg1"=0.0, "freq1"=0.0, "freq2"=0.0}, "Start following 1"=FALSE, "Start following 2"=FALSE}} ("Cluster"), "Info.Resource"="AFE_Forming", "Info.Problem"=w174, "Info.Timestamp"=w162, "Data.Forming/Following"=w170, "Data.measurements"=w164, "Data.Status"=w169) -> (w176:T11)
    n116 = Flatten To JSON(anything=w176, error in (no error)=w153) -> (JSON string=w159:string, 11:w160:errorcluster)  [unwired: 1 in]
    n117 = UDP Write(address=w154, port or service name=w155, connection ID=w152, data in=w159, 8:w160, 9:5000 ("timeout ms (25000)")) -> (error out=w156:errorcluster, 3:w151:refnum<k16>)
    n118 = local read "main stop"() -> (w150:bool)
  }
  n119 = while {
    tunnel: w25 -> [w181]
    tunnel: [w182] -> w20
    shift-right: [w183] -> _
    shift-left: T1 {"Synchronized?"=FALSE, "Sync Loss Count in"=0, "Current Sync Duration"=0} ("Status In") -> [w184]
    tunnel: w23 -> [w185]
    tunnel: "Loop Time" -> [w178]
    tunnel: [w180] -> w21
    stop <- w177 stop-if-true
    # "Run in parallel with \nyour other loops"
    # "Check Time Synch"
    n120 = Wait (ms)(milliseconds to wait=w178) -> ()  [unwired: 1 out]
    n121 = call "PM_Synch_Monitor.vi"("Polling Interval"=w178, "error in"=w181, "Status In"=w184, "Synch In"=w185) -> ("error out"=w182:errorcluster, "Status Out"=w183:T1, "Reference out"=w180:refnum<k15>, "Offset from TR (ns)"=→"Offset from TR (ns)":dbl)  [unwired: 3 in, 1 out]
    "Status Out" <- w183
    n122 = local read "main stop"() -> (w177:bool)
  }
  n123 = timed-loop {
    tunnel: w44 -> [w225]
    tunnel: [w224] -> w47
    timing: w38 -> [_]
    timing-out: [_] -> w37
    stop <- "main stop" stop-if-true
    # "WRITE CAN TO CONVERTER"
    n124 = node-c288() -> ()  [unwired: 1 in, 1 out]
    n125 = Build Array("Clear 1", "Shutdwn 1", "Emergency 1", "To IN OP 1", "SEND sp 1", "To ACT CH 1") -> (w200:bool[])
    n126 = Build Array("Clear 2", "Shutdwn 2", "Emergency 2", "To IN OP  2", "SEND sp 2", "To ACT CH 2") -> (w199:bool[])
    n127 = Build Array("Clear 3", "Shutdwn 3", "Emergency 3", "To IN OP  3", "SEND sp 3", "To ACT CH 3") -> (w198:bool[])
    n128 = Build Array("Clear 4", "Shutdwn 4", "Emergency 4", "To IN OP  4", "SEND sp 4", "To ACT CH 4") -> (w197:bool[])
    n129 = Build Array("Start forming 1", "Start following 1") -> (w191:bool[])
    n130 = Insert Into Array(array=w200, new element #1=w199, new element #2=w198, new element #3=w197, new element #4=w191) -> (w196:bool[])  [unwired: 1 in]
    n131 = Search 1D Array(1D array=w196, element=TRUE) -> (index of element=w218:i32)  [unwired: 1 in]
    n132 = Initialize Array(u8 0, 8 ("dimension size")) -> (w226:u8[])
    n133 = To Unsigned Byte Integer(number=w218) -> (unsigned 8bit integer=w222:u8)
    n134 = case shown="10" w222 {
      tunnel: w226 -> [w242 w252 w262 w273 _ w335 w345 w355 w365 w376 _ w412 w422 w432 w442 w453 _ w487 w497 w507 w517 w528 _ w558 w570 w584 w586]
      tunnel: [TRUE TRUE TRUE TRUE w324 TRUE TRUE TRUE TRUE TRUE w400 TRUE TRUE TRUE TRUE TRUE w475 TRUE TRUE TRUE TRUE TRUE w545 TRUE w561 TRUE FALSE] -> w190
      tunnel: [w234 w246 w254 w265 w291 w328 w337 w348 w357 w368 w395 w405 w414 w424 w434 w445 w469 w478 w491 w501 w511 w520 w540 w549 w563 w576 w588] -> w189
      frame 0 {
        n135 = local write "Clear 1"(FALSE ("Clear")) -> ()
        n136 = Replace Array Subset(array=w242, new element=u8 40 ("new element/subarray"), index=1) -> (w236:u8[])
        n137 = Bundle By Name(cluster=T2 {"timestamp"=timestamp(0 s since 1904-01-01), "payload"=[], "identifier"=0, "type"=0, "extended?"=FALSE, "echo?"=FALSE} ("CAN frame 3"), "payload"=w236, "identifier"=u32 24) -> (w237:T2)
        n138 = Build Array(w237) -> (w234:T2[])
      }
      frame 1 {
        n139 = local write "Shutdwn 1"(FALSE ("Shutdwn")) -> ()
        n140 = Replace Array Subset(array=w252, new element=u8 20 ("new element/subarray"), index=0) -> (w245:u8[])
        n141 = Bundle By Name(cluster=T2 {"timestamp"=timestamp(0 s since 1904-01-01), "payload"=[], "identifier"=0, "type"=0, "extended?"=FALSE, "echo?"=FALSE} ("CAN frame 3"), "payload"=w245, "identifier"=u32 24) -> (w247:T2)
        n142 = Build Array(w247) -> (w246:T2[])
      }
      frame 2 {
        n143 = local write "Emergency 1"(FALSE ("Idc cmd")) -> ()
        n144 = Replace Array Subset(array=w262, new element=u8 30 ("new element/subarray"), index=0) -> (w256:u8[])
        n145 = Bundle By Name(cluster=T2 {"timestamp"=timestamp(0 s since 1904-01-01), "payload"=[], "identifier"=0, "type"=0, "extended?"=FALSE, "echo?"=FALSE} ("CAN frame 3"), "payload"=w256, "identifier"=u32 24) -> (w257:T2)
        n146 = Build Array(w257) -> (w254:T2[])
      }
      frame 3 {
        n147 = local write "SEND sp 1"(TRUE ("SEND sp 1")) -> ()
        n148 = local write "To IN OP 1"(FALSE ("Idc cmd")) -> ()
        n149 = Replace Array Subset(array=w273, new element=u8 2 ("new element/subarray"), index=0) -> (w266:u8[])
        n150 = Bundle By Name(cluster=T2 {"timestamp"=timestamp(0 s since 1904-01-01), "payload"=[], "identifier"=0, "type"=0, "extended?"=FALSE, "echo?"=FALSE} ("CAN frame 3"), "payload"=w266, "identifier"=u32 24) -> (w268:T2)
        n151 = Build Array(w268) -> (w265:T2[])
      }
      frame 4 {
        (unwired) TRUE
        # "anlge"
        # "mag"
        # "Vdc Q mode"
        n152 = Square Root(x=2.0) -> (sqrt(x)=w290:dbl)
        n153 = Add(x="Vabs 1", y="delta V") -> (x+y=w282:dbl)
        n154 = Multiply(x=0.9861, y="Qac1") -> (x*y=w277:dbl)
        n155 = Compound Arithmetic op=MULTIPLY(100.0 ("value"), w290, w282) -> (w288:dbl)
        n156 = local write "SEND sp 1"(FALSE ("SEND sp")) -> ()
        n157 = Multiply(x=10000.0, y="Varg 1") -> (x*y=w300:dbl)
        n158 = Add(x=w277, y=44.8 ("biasP2")) -> (x+y=w276:dbl)
        n159 = Add(x="Vdc1", y="biasV1") -> (x+y=w286:dbl)
        n160 = To Unsigned Word Integer(number=w288) -> (unsigned 16bit integer=w305:u16)
        n161 = To Word Integer(number=w300) -> (16bit integer=w301:i16)
        n162 = Add(x="freq 1", y="delta f") -> (x+y=w284:dbl)
        n163 = call "Vdc_lim.vi"("IN Vdc"=w286) -> ("OUT Vdc"=w316:dbl)  [unwired: 10 in]
        n164 = call "Q_limiter.vi"("IN Q"=w276) -> ("OUT Q"=w315:dbl)  [unwired: 10 in]
        n165 = Split Number(x=w305) -> (hi(x)=w306:u8, lo(x)=w307:u8)
        n166 = Split Number(x=w301) -> (hi(x)=w302:u8, lo(x)=w303:u8)
        n167 = Build Array(w306, w307) -> (w308:u8[])
        n168 = call "DoubleToSetpoint.vi"("Double"=w316) -> ("SP"=w318:u8[])
        n169 = call "DoubleToSetpoint.vi"("Double"=w315) -> ("SP"=w317:u8[])
        n170 = Build Array(w302, w303) -> (w304:u8[])
        n171 = Multiply(x=100000.0, y=w284) -> (x*y=w310:dbl)
        n172 = Reverse 1D Array(array=w308) -> (reversed array=w299:u8[])
        n173 = call "DoubleToSetpoint.vi"("Double"=w310) -> ("SP"=w297:u8[])
        n174 = Reverse 1D Array(array=w304) -> (reversed array=w298:u8[])
        n175 = Build Array (concatenate)(w318, w317) -> (w320:u8[])
        n176 = Build Array (concatenate)(w299, w298, w297) -> (w295:u8[])
        n177 = Bundle By Name(cluster=T2 {"timestamp"=timestamp(0 s since 1904-01-01), "payload"=[], "identifier"=0, "type"=0, "extended?"=FALSE, "echo?"=FALSE} ("CAN frame 3"), "payload"=w295, "identifier"=u32 20) -> (w292:T2)
        n178 = Bundle By Name(cluster=T2 {"timestamp"=timestamp(0 s since 1904-01-01), "payload"=[], "identifier"=0, "type"=0, "extended?"=FALSE, "echo?"=FALSE} ("CAN frame 3"), "payload"=w320, "identifier"=u32 19) -> (w293:T2)
        n179 = Build Array(w292, w293) -> (w291:T2[])
        n180 = Build Array(w292) -> ()  [unwired: 1 out]
        n181 = local read "Ready 1"() -> (w322:bool)
        n182 = local read "ON 1"() -> (w323:bool)
        n183 = Or(x=w323, y=w322) -> (x .or. y?=w324:bool)
      }
      frame 5 {
        n184 = local write "To ACT CH 1"(FALSE ("Idc cmd")) -> ()
        n185 = local write "SEND sp 1"(TRUE ("SEND sp 1")) -> ()
        n186 = Replace Array Subset(array=w335, new element=u8 1 ("new element/subarray"), index=0) -> (w327:u8[])
        n187 = Bundle By Name(cluster=T2 {"timestamp"=timestamp(0 s since 1904-01-01), "payload"=[], "identifier"=0, "type"=0, "extended?"=FALSE, "echo?"=FALSE} ("CAN frame 3"), "payload"=w327, "identifier"=u32 24) -> (w329:T2)
        n188 = Build Array(w329) -> (w328:T2[])
      }
      frame 6 {
        n189 = local write "Clear 2"(FALSE ("Clear")) -> ()
        n190 = Replace Array Subset(array=w345, new element=u8 40 ("new element/subarray"), index=1) -> (w339:u8[])
        n191 = Bundle By Name(cluster=T2 {"timestamp"=timestamp(0 s since 1904-01-01), "payload"=[], "identifier"=0, "type"=0, "extended?"=FALSE, "echo?"=FALSE} ("CAN frame 3"), "payload"=w339, "identifier"=u32 40) -> (w340:T2)
        n192 = Build Array(w340) -> (w337:T2[])
      }
      frame 7 {
        n193 = local write "Shutdwn 2"(FALSE ("Shutdwn")) -> ()
        n194 = Replace Array Subset(array=w355, new element=u8 20 ("new element/subarray"), index=0) -> (w349:u8[])
        n195 = Bundle By Name(cluster=T2 {"timestamp"=timestamp(0 s since 1904-01-01), "payload"=[], "identifier"=0, "type"=0, "extended?"=FALSE, "echo?"=FALSE} ("CAN frame 3"), "payload"=w349, "identifier"=u32 40) -> (w350:T2)
        n196 = Build Array(w350) -> (w348:T2[])
      }
      frame 8 {
        n197 = local write "Emergency 2"(FALSE ("Idc cmd")) -> ()
        n198 = Replace Array Subset(array=w365, new element=u8 30 ("new element/subarray"), index=0) -> (w359:u8[])
        n199 = Bundle By Name(cluster=T2 {"timestamp"=timestamp(0 s since 1904-01-01), "payload"=[], "identifier"=0, "type"=0, "extended?"=FALSE, "echo?"=FALSE} ("CAN frame 3"), "payload"=w359, "identifier"=u32 40) -> (w360:T2)
        n200 = Build Array(w360) -> (w357:T2[])
      }
      frame 9 {
        n201 = local write "SEND sp 2"(TRUE ("SEND sp 2")) -> ()
        n202 = local write "To IN OP  2"(FALSE ("Idc cmd")) -> ()
        n203 = Replace Array Subset(array=w376, new element=u8 2 ("new element/subarray"), index=0) -> (w370:u8[])
        n204 = Bundle By Name(cluster=T2 {"timestamp"=timestamp(0 s since 1904-01-01), "payload"=[], "identifier"=0, "type"=0, "extended?"=FALSE, "echo?"=FALSE} ("CAN frame 3"), "payload"=w370, "identifier"=u32 40) -> (w371:T2)
        n205 = Build Array(w371) -> (w368:T2[])
      }
      frame 10 {
        # "Vdc Q mode"
        n206 = Multiply(x=1.24797, y="Pac2") -> (x*y=w385:dbl)
        n207 = Multiply(x=1.2802, y="Qac2") -> (x*y=w382:dbl)
        n208 = Add(x=w385, y=1787.9 ("biasP2")) -> (x+y=w386:dbl)
        n209 = Add(x=w382, y=203.7 ("biasP2")) -> (x+y=w379:dbl)
        n210 = Add(x=w379, y="Q2 bias") -> (x+y=w378:dbl)
        n211 = call "Q_limiter.vi"("IN Q"=w386) -> ("OUT Q"=w389:dbl)  [unwired: 10 in]
        n212 = call "Q_limiter.vi"("IN Q"=w378) -> ("OUT Q"=w392:dbl)  [unwired: 10 in]
        n213 = call "DoubleToSetpoint.vi"("Double"=w389) -> ("SP"=w394:u8[])
        n214 = call "DoubleToSetpoint.vi"("Double"=w392) -> ("SP"=w393:u8[])
        n215 = Build Array (concatenate)(w394, w393) -> (w397:u8[])
        n216 = local write "SEND sp 2"(FALSE ("SEND sp 2")) -> ()
        n217 = Bundle By Name(cluster=T2 {"timestamp"=timestamp(0 s since 1904-01-01), "payload"=[], "identifier"=0, "type"=0, "extended?"=FALSE, "echo?"=FALSE} ("CAN frame 3"), "payload"=w397, "identifier"=u32 35) -> (w398:T2)
        n218 = Build Array(w398) -> (w395:T2[])
        n219 = local read "ON 2"() -> (w401:bool)
        n220 = local read "Ready 2"() -> (w402:bool)
        n221 = Or(x=w401, y=w402) -> (x .or. y?=w400:bool)
      }
      frame 11 {
        n222 = local write "To ACT CH 2"(FALSE ("Idc cmd")) -> ()
        n223 = local write "SEND sp 2"(TRUE ("SEND sp 2")) -> ()
        n224 = Replace Array Subset(array=w412, new element=u8 1 ("new element/subarray"), index=0) -> (w404:u8[])
        n225 = Bundle By Name(cluster=T2 {"timestamp"=timestamp(0 s since 1904-01-01), "payload"=[], "identifier"=0, "type"=0, "extended?"=FALSE, "echo?"=FALSE} ("CAN frame 3"), "payload"=w404, "identifier"=u32 40) -> (w406:T2)
        n226 = Build Array(w406) -> (w405:T2[])
      }
      frame 12 {
        n227 = local write "Clear 3"(FALSE ("Clear")) -> ()
        n228 = Replace Array Subset(array=w422, new element=u8 40 ("new element/subarray"), index=1) -> (w416:u8[])
        n229 = Bundle By Name(cluster=T2 {"timestamp"=timestamp(0 s since 1904-01-01), "payload"=[], "identifier"=0, "type"=0, "extended?"=FALSE, "echo?"=FALSE} ("CAN frame 3"), "payload"=w416, "identifier"=u32 56) -> (w417:T2)
        n230 = Build Array(w417) -> (w414:T2[])
      }
      frame 13 {
        n231 = local write "Shutdwn 3"(FALSE ("Shutdwn")) -> ()
        n232 = Replace Array Subset(array=w432, new element=u8 20 ("new element/subarray"), index=0) -> (w426:u8[])
        n233 = Bundle By Name(cluster=T2 {"timestamp"=timestamp(0 s since 1904-01-01), "payload"=[], "identifier"=0, "type"=0, "extended?"=FALSE, "echo?"=FALSE} ("CAN frame 3"), "payload"=w426, "identifier"=u32 56) -> (w427:T2)
        n234 = Build Array(w427) -> (w424:T2[])
      }
      frame 14 {
        n235 = local write "Emergency 3"(FALSE ("Idc cmd")) -> ()
        n236 = Replace Array Subset(array=w442, new element=u8 30 ("new element/subarray"), index=0) -> (w436:u8[])
        n237 = Bundle By Name(cluster=T2 {"timestamp"=timestamp(0 s since 1904-01-01), "payload"=[], "identifier"=0, "type"=0, "extended?"=FALSE, "echo?"=FALSE} ("CAN frame 3"), "payload"=w436, "identifier"=u32 56) -> (w437:T2)
        n238 = Build Array(w437) -> (w434:T2[])
      }
      frame 15 {
        n239 = local write "SEND sp 3"(TRUE ("SEND sp 3")) -> ()
        n240 = local write "To IN OP  3"(FALSE ("Idc cmd")) -> ()
        n241 = Replace Array Subset(array=w453, new element=u8 2 ("new element/subarray"), index=0) -> (w447:u8[])
        n242 = Bundle By Name(cluster=T2 {"timestamp"=timestamp(0 s since 1904-01-01), "payload"=[], "identifier"=0, "type"=0, "extended?"=FALSE, "echo?"=FALSE} ("CAN frame 3"), "payload"=w447, "identifier"=u32 56) -> (w448:T2)
        n243 = Build Array(w448) -> (w445:T2[])
      }
      frame 16 {
        # "Vdc Q mode"
        n244 = Multiply(x=0.9759, y="Pac3") -> (x*y=w462:dbl)
        n245 = Multiply(x=0.9903, y="Qac3") -> (x*y=w459:dbl)
        n246 = local write "SEND sp 3"(FALSE ("SEND sp")) -> ()
        n247 = Add(x=w462, y=1396.4 ("biasP2")) -> (x+y=w456:dbl)
        n248 = Add(x=w459, y=102.6 ("biasP2")) -> (x+y=w455:dbl)
        n249 = call "Q_limiter.vi"("IN Q"=w456) -> ("OUT Q"=w465:dbl)  [unwired: 10 in]
        n250 = call "Q_limiter.vi"("IN Q"=w455) -> ("OUT Q"=w466:dbl)  [unwired: 10 in]
        n251 = call "DoubleToSetpoint.vi"("Double"=w465) -> ("SP"=w468:u8[])
        n252 = call "DoubleToSetpoint.vi"("Double"=w466) -> ("SP"=w467:u8[])
        n253 = Build Array (concatenate)(w468, w467) -> (w471:u8[])
        n254 = local read "ON 3"() -> (w476:bool)
        n255 = local read "Ready 3"() -> (w474:bool)
        n256 = Or(x=w476, y=w474) -> (x .or. y?=w475:bool)
        n257 = Bundle By Name(cluster=T2 {"timestamp"=timestamp(0 s since 1904-01-01), "payload"=[], "identifier"=0, "type"=0, "extended?"=FALSE, "echo?"=FALSE} ("CAN frame 3"), "payload"=w471, "identifier"=u32 51) -> (w472:T2)
        n258 = Build Array(w472) -> (w469:T2[])
      }
      frame 17 {
        n259 = local write "To ACT CH 3"(FALSE ("Idc cmd")) -> ()
        n260 = local write "SEND sp 3"(TRUE ("SEND sp 3")) -> ()
        n261 = Replace Array Subset(array=w487, new element=u8 1 ("new element/subarray"), index=0) -> (w480:u8[])
        n262 = Bundle By Name(cluster=T2 {"timestamp"=timestamp(0 s since 1904-01-01), "payload"=[], "identifier"=0, "type"=0, "extended?"=FALSE, "echo?"=FALSE} ("CAN frame 3"), "payload"=w480, "identifier"=u32 56) -> (w481:T2)
        n263 = Build Array(w481) -> (w478:T2[])
      }
      frame 18 {
        n264 = local write "Clear 4"(FALSE ("Clear")) -> ()
        n265 = Replace Array Subset(array=w497, new element=u8 40 ("new element/subarray"), index=1) -> (w490:u8[])
        n266 = Bundle By Name(cluster=T2 {"timestamp"=timestamp(0 s since 1904-01-01), "payload"=[], "identifier"=0, "type"=0, "extended?"=FALSE, "echo?"=FALSE} ("CAN frame 3"), "payload"=w490, "identifier"=u32 72) -> (w492:T2)
        n267 = Build Array(w492) -> (w491:T2[])
      }
      frame 19 {
        n268 = local write "Shutdwn 4"(FALSE ("Shutdwn")) -> ()
        n269 = Replace Array Subset(array=w507, new element=u8 20 ("new element/subarray"), index=0) -> (w500:u8[])
        n270 = Bundle By Name(cluster=T2 {"timestamp"=timestamp(0 s since 1904-01-01), "payload"=[], "identifier"=0, "type"=0, "extended?"=FALSE, "echo?"=FALSE} ("CAN frame 3"), "payload"=w500, "identifier"=u32 72) -> (w502:T2)
        n271 = Build Array(w502) -> (w501:T2[])
      }
      frame 20 {
        n272 = local write "Emergency 4"(FALSE ("Idc cmd")) -> ()
        n273 = Replace Array Subset(array=w517, new element=u8 30 ("new element/subarray"), index=0) -> (w510:u8[])
        n274 = Bundle By Name(cluster=T2 {"timestamp"=timestamp(0 s since 1904-01-01), "payload"=[], "identifier"=0, "type"=0, "extended?"=FALSE, "echo?"=FALSE} ("CAN frame 3"), "payload"=w510, "identifier"=u32 72) -> (w512:T2)
        n275 = Build Array(w512) -> (w511:T2[])
      }
      frame 21 {
        n276 = local write "SEND sp 4"(TRUE ("SEND sp 4")) -> ()
        n277 = local write "To IN OP  4"(FALSE ("Idc cmd")) -> ()
        n278 = Replace Array Subset(array=w528, new element=u8 2 ("new element/subarray"), index=0) -> (w522:u8[])
        n279 = Bundle By Name(cluster=T2 {"timestamp"=timestamp(0 s since 1904-01-01), "payload"=[], "identifier"=0, "type"=0, "extended?"=FALSE, "echo?"=FALSE} ("CAN frame 3"), "payload"=w522, "identifier"=u32 72) -> (w523:T2)
        n280 = Build Array(w523) -> (w520:T2[])
      }
      frame 22 {
        # "Vdc Q mode"
        n281 = Add(x="Qac4", y="biasQ4") -> (x+y=w530:dbl)
        n282 = local write "SEND sp 4"(FALSE ("SEND sp")) -> ()
        n283 = Add(x="Vdc4", y="biasV4") -> (x+y=w534:dbl)
        n284 = call "Q_limiter.vi"("IN Q"=w530) -> ("OUT Q"=w536:dbl)  [unwired: 10 in]
        n285 = call "Vdc_lim.vi"("IN Vdc"=w534) -> ("OUT Vdc"=w537:dbl)  [unwired: 10 in]
        n286 = call "DoubleToSetpoint.vi"("Double"=w537) -> ("SP"=w539:u8[])
        n287 = call "DoubleToSetpoint.vi"("Double"=w536) -> ("SP"=w538:u8[])
        n288 = Build Array (concatenate)(w539, w538) -> (w542:u8[])
        n289 = local read "ON 4"() -> (w546:bool)
        n290 = local read "Ready 4"() -> (w547:bool)
        n291 = Or(x=w546, y=w547) -> (x .or. y?=w545:bool)
        n292 = Bundle By Name(cluster=T2 {"timestamp"=timestamp(0 s since 1904-01-01), "payload"=[], "identifier"=0, "type"=0, "extended?"=FALSE, "echo?"=FALSE} ("CAN frame 3"), "payload"=w542, "identifier"=u32 67) -> (w543:T2)
        n293 = Build Array(w543) -> (w540:T2[])
      }
      frame 23 {
        n294 = local write "To ACT CH 4"(FALSE ("Idc cmd")) -> ()
        n295 = local write "SEND sp 4"(TRUE ("SEND sp 4")) -> ()
        n296 = Replace Array Subset(array=w558, new element=u8 1 ("new element/subarray"), index=0) -> (w551:u8[])
        n297 = Bundle By Name(cluster=T2 {"timestamp"=timestamp(0 s since 1904-01-01), "payload"=[], "identifier"=0, "type"=0, "extended?"=FALSE, "echo?"=FALSE} ("CAN frame 3"), "payload"=w551, "identifier"=u32 72) -> (w552:T2)
        n298 = Build Array(w552) -> (w549:T2[])
      }
      frame 24 {
        # "it take on average 500ms to close the switch\n-> therefore, we wait 200ms so the converter is only following in grid connected mode for 300ms\n-> this guarentees a more smooth stransition"
        # "start forming 1"
        n299 = local write "Start forming 1"(FALSE ("Start following 1")) -> ()
        n300 = local write "SEND sp 1"(TRUE ("SEND sp 1")) -> ()
        n301 = Replace Array Subset(array=w570, new element=u8 3 ("new element/subarray"), index=0) -> (w565:u8[])
        n302 = flat-sequence {
          tunnel: [TRUE] -> w560
          tunnel: [w574] -> w561
          tunnel: w560 -> [w574]
          frame #0 {
          }
          frame #1 {
            # "40"
            n303 = Wait (ms)(milliseconds to wait=u32 80) -> ()  [unwired: 1 out]
          }
        }
        n304 = Bundle By Name(cluster=T2 {"timestamp"=timestamp(0 s since 1904-01-01), "payload"=[], "identifier"=0, "type"=0, "extended?"=FALSE, "echo?"=FALSE} ("CAN frame 3"), "payload"=w565, "identifier"=u32 24) -> (w566:T2)
        n305 = Build Array(w566) -> (w563:T2[])
      }
      frame 25 {
        # "it take on average 140ms to open the switch\n-> to be sure the grid is connected before we stors following, we add a 300ms delay\n-> the converter can easily sustain 160ms in forming mode when grid connected"
        # "start following 1"
        n306 = local write "Start following 1"(FALSE ("Start forming 1")) -> ()
        n307 = local write "SEND sp 1"(TRUE ("SEND sp 1")) -> ()
        n308 = Replace Array Subset(array=w584, new element=u8 2 ("new element/subarray"), index=0) -> (w578:u8[])
        n309 = Bundle By Name(cluster=T2 {"timestamp"=timestamp(0 s since 1904-01-01), "payload"=[], "identifier"=0, "type"=0, "extended?"=FALSE, "echo?"=FALSE} ("CAN frame 3"), "payload"=w578, "identifier"=u32 24) -> (w579:T2)
        n310 = Build Array(w579) -> (w576:T2[])
      }
      frame 99, Default {
        n311 = Bundle By Name(cluster=T2 {"timestamp"=timestamp(0 s since 1904-01-01), "payload"=[], "identifier"=0, "type"=0, "extended?"=FALSE, "echo?"=FALSE} ("CAN frame 3"), "payload"=w586, "identifier"=u32 18) -> (w589:T2)
        n312 = Build Array(w589) -> (w588:T2[])
      }
    }
    n313 = case shown="True" w190 {
      tunnel: w189 -> [w231 _]
      tunnel: w225 -> [w233 _]
      tunnel: [w232 _] -> w224
      frame True {
        n314 = call-poly <vilib>:"XNET Write.vi"("session in"=w233, "data"=w231) -> ("session out"=w232:refnum<k21>)  [unwired: 12 in, 1 out]
        "CAN OUT" <- w231
      }
      frame False {
      }
    }
    n315 = node-c288() -> ()  [unwired: 1 in, 1 out]
  }
  n316 = timed-loop {
    timing: w43 -> [_]
    timing-out: [_] -> w42
    tunnel: w41 -> [w595]
    tunnel: [w601] -> w48
    shift-right: [w596] -> _
    shift-left: T6 {"State 1"=4.0, "code 1"=0.0, "code 2"=0.0, "code 3"=0.0, "code 4"=0.0, "State 2"=4.0, "State 3"=4.0, "State 4"=4.0} ("Conv 2") -> [w600]
    tunnel: [FALSE ("stop CAN")] -> w45
    shift-right: [w593] -> _
    shift-left: T4 {"Vdc1"=0.0, "P1"=0.0, "Vdc2"=0.0, "P2"=0.0, "Q2"=0.0, "Vdc3"=0.0, "P3"=0.0, "Q3"=0.0, "Vdc4"=0.0, "P4"=0.0, "Q4"=0.0, "Q1"=0.0} ("measurements 2") -> [w594]
    stop <- w599 stop-if-true
    # "state 21: forming, state 23 is following"
    # "READ CAN FROM CONVERTER"
    n317 = node-c288() -> ()  [unwired: 1 in, 1 out]
    n318 = local write "CAN with Conv"(TRUE) -> ()
    n319 = call-poly <vilib>:"XNET Read.vi"("session in"=w595) -> ("session out"=w601:refnum<k21>, "data"=w602:T2[])  [unwired: 11 in, 2 out]
    n320 = Get Date/Time In Seconds() -> (seconds since 1Jan1904=→"current time":timestamp)
    n321 = for {
      tunnel: w602 -> [w607] mode=indexing
      shift-right: [w605] -> w596
      shift-left: w600 -> [w606]
      shift-right: [w603] -> w593
      shift-left: w594 -> [w604]
      n322 = Unbundle By Name(w607) -> ("identifier"=w609:u32, "payload"=w608:u8[])
      n323 = case shown="102" w609 {
        tunnel: w608 -> [_ w616 w650 w675 w700 w727 w734 w741 w748 w753 w761 w769 w777]
        tunnel: w606 -> [w611 w624 w658 w683 w708 w725 w732 w739 w746 w751 w757 w766 w774]
        tunnel: [w611 w623 w657 w682 w707 w725 w732 w739 w746 w751 w757 w766 w774] -> w605
        tunnel: w604 -> [w610 w613 w647 w672 w698 w723 w728 w735 w742 w749 w756 w765 w772]
        tunnel: [w610 w614 w648 w673 w699 w724 w729 w736 w743 w750 w755 w764 w773] -> w603
        frame 0, Default {
        }
        frame 25 {
          w612 = 1.0 ("factor 1")
          n324 = Index Array(array=w616, index=0) -> (element=w617:u8)
          n325 = call "U8arrayToMeasurement.vi"("factor 2"=w612, "factor 1"=w612, "payload"=w616) -> ("Meas 2"=w615:dbl)  [unwired: 1 out]
          "V slider 19" <- w615
          n326 = Index Array(array=w616, index=1) -> (element=w620:u8)
          n327 = Index Array(array=w616, index=2) -> (element=w619:u8)
          n328 = Join Numbers(hi=w620, lo=w619) -> ((hi.lo)=w618:u16)
          "State code 1" <- w618
          n329 = Bundle By Name(cluster=w613, "Vdc1"=w615) -> (w614:T4)
          n330 = case shown="5" w617 {
            frame 5 {
              w627 = FALSE ("Fault 1")
              n331 = local write "Forming 1"(FALSE ("Forming 1")) -> ()
              n332 = local write "Fault 1"(TRUE ("Fault 1")) -> ()
              n333 = local write "Error 1"(w627) -> ()
              n334 = local write "OFF 1"(w627) -> ()
              n335 = local write "Ready 1"(w627) -> ()
              n336 = local write "ON 1"(w627) -> ()
            }
            frame 6 {
              w631 = FALSE ("Fault 1")
              n337 = local write "Fault 1"(w631) -> ()
              n338 = local write "Error 1"(w631) -> ()
              n339 = local write "OFF 1"(w631) -> ()
              n340 = local write "Ready 1"(w631) -> ()
              n341 = local write "ON 1"(TRUE ("Fault 1")) -> ()
              n342 = local write "Forming 1"(TRUE ("Forming 1")) -> ()
            }
            frame 1 {
              w633 = FALSE ("Fault 1")
              n343 = local write "Forming 1"(FALSE ("Forming 1")) -> ()
              n344 = local write "Fault 1"(w633) -> ()
              n345 = local write "Error 1"(TRUE ("Error 1")) -> ()
              n346 = local write "OFF 1"(w633) -> ()
              n347 = local write "Ready 1"(w633) -> ()
              n348 = local write "ON 1"(w633) -> ()
            }
            frame 2 {
              w637 = FALSE ("Fault 1")
              n349 = local write "Forming 1"(FALSE ("Forming 1")) -> ()
              n350 = local write "Fault 1"(w637) -> ()
              n351 = local write "Error 1"(w637) -> ()
              n352 = local write "OFF 1"(TRUE ("OFF 1")) -> ()
              n353 = local write "Ready 1"(w637) -> ()
              n354 = local write "ON 1"(w637) -> ()
            }
            frame 3 {
              w640 = FALSE ("Fault 1")
              n355 = local write "Forming 1"(FALSE ("Forming 1")) -> ()
              n356 = local write "Fault 1"(w640) -> ()
              n357 = local write "Error 1"(w640) -> ()
              n358 = local write "OFF 1"(w640) -> ()
              n359 = local write "Ready 1"(TRUE ("Ready 1")) -> ()
              n360 = local write "ON 1"(w640) -> ()
            }
            frame 4 {
              w643 = FALSE ("Fault 1")
              n361 = local write "Fault 1"(w643) -> ()
              n362 = local write "Error 1"(w643) -> ()
              n363 = local write "OFF 1"(w643) -> ()
              n364 = local write "Ready 1"(w643) -> ()
              n365 = local write "Forming 1"(FALSE ("Forming 1")) -> ()
              n366 = local write "ON 1"(TRUE ("ON 1")) -> ()
            }
            frame 99, Default {
              w645 = FALSE ("Fault 1")
              n367 = local write "Forming 1"(FALSE ("Forming 1")) -> ()
              n368 = local write "Fault 1"(w645) -> ()
              n369 = local write "Error 1"(w645) -> ()
              n370 = local write "OFF 1"(w645) -> ()
              n371 = local write "Ready 1"(w645) -> ()
              n372 = local write "ON 1"(w645) -> ()
            }
          }
          n373 = Bundle By Name(cluster=w624, "State 1"=w617, "code 1"=w618) -> (w623:T6)
        }
        frame 41 {
          w646 = 1.0 ("factor 1")
          n374 = call "U8arrayToMeasurement.vi"("factor 2"=w646, "factor 1"=w646, "payload"=w650) -> ("Meas 2"=w649:dbl)  [unwired: 1 out]
          "V slider 20" <- w649
          n375 = Index Array(array=w650, index=0) -> (element=w656:u8)
          n376 = Index Array(array=w650, index=1) -> (element=w653:u8)
          n377 = Index Array(array=w650, index=2) -> (element=w652:u8)
          n378 = Join Numbers(hi=w653, lo=w652) -> ((hi.lo)=w651:u16)
          "State code 2" <- w651
          n379 = Bundle By Name(cluster=w647, "Vdc2"=w649) -> (w648:T4)
          n380 = case shown="5" w656 {
            frame 5 {
              w661 = FALSE ("Fault 1")
              n381 = local write "Fault 2"(TRUE ("Fault 1")) -> ()
              n382 = local write "Error 2"(w661) -> ()
              n383 = local write "OFF 2"(w661) -> ()
              n384 = local write "Ready 2"(w661) -> ()
              n385 = local write "ON 2"(w661) -> ()
            }
            frame 1 {
              w662 = FALSE ("Fault 1")
              n386 = local write "Fault 2"(w662) -> ()
              n387 = local write "Error 2"(TRUE ("Error 1")) -> ()
              n388 = local write "OFF 2"(w662) -> ()
              n389 = local write "Ready 2"(w662) -> ()
              n390 = local write "ON 2"(w662) -> ()
            }
            frame 2 {
              w665 = FALSE ("Fault 1")
              n391 = local write "Fault 2"(w665) -> ()
              n392 = local write "Error 2"(w665) -> ()
              n393 = local write "OFF 2"(TRUE ("OFF 1")) -> ()
              n394 = local write "Ready 2"(w665) -> ()
              n395 = local write "ON 2"(w665) -> ()
            }
            frame 3 {
              w667 = FALSE ("Fault 1")
              n396 = local write "Fault 2"(w667) -> ()
              n397 = local write "Error 2"(w667) -> ()
              n398 = local write "OFF 2"(w667) -> ()
              n399 = local write "Ready 2"(TRUE ("Ready 1")) -> ()
              n400 = local write "ON 2"(w667) -> ()
            }
            frame 4 {
              w669 = FALSE ("Fault 1")
              n401 = local write "Fault 2"(w669) -> ()
              n402 = local write "Error 2"(w669) -> ()
              n403 = local write "OFF 2"(w669) -> ()
              n404 = local write "Ready 2"(w669) -> ()
              n405 = local write "ON 2"(TRUE ("ON 1")) -> ()
            }
            frame 99, Default {
              w670 = FALSE ("Fault 1")
              n406 = local write "Fault 2"(w670) -> ()
              n407 = local write "Error 2"(w670) -> ()
              n408 = local write "OFF 2"(w670) -> ()
              n409 = local write "Ready 2"(w670) -> ()
              n410 = local write "ON 2"(w670) -> ()
            }
          }
          n411 = Bundle By Name(cluster=w658, "State 2"=w656, "code 2"=w651) -> (w657:T6)
        }
        frame 57 {
          w671 = 1.0 ("factor 1")
          n412 = Index Array(array=w675, index=0) -> (element=w681:u8)
          n413 = Index Array(array=w675, index=1) -> (element=w678:u8)
          n414 = Index Array(array=w675, index=2) -> (element=w677:u8)
          n415 = call "U8arrayToMeasurement.vi"("factor 2"=w671, "factor 1"=w671, "payload"=w675) -> ("Meas 2"=w674:dbl)  [unwired: 1 out]
          "V slider 21" <- w674
          n416 = Join Numbers(hi=w678, lo=w677) -> ((hi.lo)=w676:u16)
          "State code 3" <- w676
          n417 = case shown="5" w681 {
            frame 5 {
              w686 = FALSE ("Fault 1")
              n418 = local write "Fault 3"(TRUE ("Fault 1")) -> ()
              n419 = local write "Error 3"(w686) -> ()
              n420 = local write "OFF 3"(w686) -> ()
              n421 = local write "Ready 3"(w686) -> ()
              n422 = local write "ON 3"(w686) -> ()
            }
            frame 1 {
              w687 = FALSE ("Fault 1")
              n423 = local write "Fault 3"(w687) -> ()
              n424 = local write "Error 3"(TRUE ("Error 1")) -> ()
              n425 = local write "OFF 3"(w687) -> ()
              n426 = local write "Ready 3"(w687) -> ()
              n427 = local write "ON 3"(w687) -> ()
            }
            frame 2 {
              w690 = FALSE ("Fault 1")
              n428 = local write "Fault 3"(w690) -> ()
              n429 = local write "Error 3"(w690) -> ()
              n430 = local write "OFF 3"(TRUE ("OFF 1")) -> ()
              n431 = local write "Ready 3"(w690) -> ()
              n432 = local write "ON 3"(w690) -> ()
            }
            frame 3 {
              w692 = FALSE ("Fault 1")
              n433 = local write "Fault 3"(w692) -> ()
              n434 = local write "Error 3"(w692) -> ()
              n435 = local write "OFF 3"(w692) -> ()
              n436 = local write "Ready 3"(TRUE ("Ready 1")) -> ()
              n437 = local write "ON 3"(w692) -> ()
            }
            frame 4 {
              w694 = FALSE ("Fault 1")
              n438 = local write "Fault 3"(w694) -> ()
              n439 = local write "Error 3"(w694) -> ()
              n440 = local write "OFF 3"(w694) -> ()
              n441 = local write "Ready 3"(w694) -> ()
              n442 = local write "ON 3"(TRUE ("ON 1")) -> ()
            }
            frame 99, Default {
              w695 = FALSE ("Fault 1")
              n443 = local write "Fault 3"(w695) -> ()
              n444 = local write "Error 3"(w695) -> ()
              n445 = local write "OFF 3"(w695) -> ()
              n446 = local write "Ready 3"(w695) -> ()
              n447 = local write "ON 3"(w695) -> ()
            }
          }
          n448 = Bundle By Name(cluster=w672, "Vdc3"=w674) -> (w673:T4)
          n449 = Bundle By Name(cluster=w683, "State 3"=w681, "code 3"=w676) -> (w682:T6)
        }
        frame 73 {
          w696 = 1.0 ("factor 1")
          n450 = Index Array(array=w700, index=0) -> (element=w706:u8)
          n451 = Index Array(array=w700, index=1) -> (element=w703:u8)
          n452 = Index Array(array=w700, index=2) -> (element=w702:u8)
          n453 = Join Numbers(hi=w703, lo=w702) -> ((hi.lo)=w701:u16)
          "State code 4" <- w701
          n454 = call "U8arrayToMeasurement.vi"("factor 2"=w696, "factor 1"=w696, "payload"=w700) -> ("Meas 2"=w697:dbl)  [unwired: 1 out]
          "V slider 22" <- w697
          n455 = case shown="5" w706 {
            frame 5 {
              w711 = FALSE ("Fault 1")
              n456 = local write "Fault 4"(TRUE ("Fault 1")) -> ()
              n457 = local write "Error 4"(w711) -> ()
              n458 = local write "OFF 4"(w711) -> ()
              n459 = local write "Ready 4"(w711) -> ()
              n460 = local write "ON 4"(w711) -> ()
            }
            frame 1 {
              w712 = FALSE ("Fault 1")
              n461 = local write "Fault 4"(w712) -> ()
              n462 = local write "Error 4"(TRUE ("Error 1")) -> ()
              n463 = local write "OFF 4"(w712) -> ()
              n464 = local write "Ready 4"(w712) -> ()
              n465 = local write "ON 4"(w712) -> ()
            }
            frame 2 {
              w715 = FALSE ("Fault 1")
              n466 = local write "Fault 4"(w715) -> ()
              n467 = local write "Error 4"(w715) -> ()
              n468 = local write "OFF 4"(TRUE ("OFF 1")) -> ()
              n469 = local write "Ready 4"(w715) -> ()
              n470 = local write "ON 4"(w715) -> ()
            }
            frame 3 {
              w717 = FALSE ("Fault 1")
              n471 = local write "Fault 4"(w717) -> ()
              n472 = local write "Error 4"(w717) -> ()
              n473 = local write "OFF 4"(w717) -> ()
              n474 = local write "Ready 4"(TRUE ("Ready 1")) -> ()
              n475 = local write "ON 4"(w717) -> ()
            }
            frame 4 {
              w719 = FALSE ("Fault 1")
              n476 = local write "Fault 4"(w719) -> ()
              n477 = local write "Error 4"(w719) -> ()
              n478 = local write "OFF 4"(w719) -> ()
              n479 = local write "Ready 4"(w719) -> ()
              n480 = local write "ON 4"(TRUE ("ON 1")) -> ()
            }
            frame 99, Default {
              w720 = FALSE ("Fault 1")
              n481 = local write "Fault 4"(w720) -> ()
              n482 = local write "Error 4"(w720) -> ()
              n483 = local write "OFF 4"(w720) -> ()
              n484 = local write "Ready 4"(w720) -> ()
              n485 = local write "ON 4"(w720) -> ()
            }
          }
          n486 = Bundle By Name(cluster=w698, "Vdc4"=w697) -> (w699:T4)
          n487 = Bundle By Name(cluster=w708, "State 4"=w706, "code 4"=w701) -> (w707:T6)
        }
        frame 258 {
          w726 = 1000.0 ("factor 1")
          # "Q"
          # "P"
          n488 = call "U8arrayToMeasurement.vi"("factor 2"=w726, "factor 1"=w726, "payload"=w727) -> ("Meas 2"=w721:dbl, "Meas 1"=w722:dbl)
          "kW" <- w722
          "?VkVAr" <- w721
          n489 = Bundle By Name(cluster=w723, "P1"=w722, "Q1"=w721) -> (w724:T4)
        }
        frame 514 {
          w733 = 1000.0 ("factor 1")
          # "Q"
          # "P"
          n490 = call "U8arrayToMeasurement.vi"("factor 2"=w733, "factor 1"=w733, "payload"=w734) -> ("Meas 2"=w730:dbl, "Meas 1"=w731:dbl)
          "kW" <- w731
          "?VkVAr" <- w730
          n491 = Bundle By Name(cluster=w728, "P2"=w731, "Q2"=w730) -> (w729:T4)
        }
        frame 770 {
          w740 = 1000.0 ("factor 1")
          # "Q"
          # "P"
          n492 = call "U8arrayToMeasurement.vi"("factor 2"=w740, "factor 1"=w740, "payload"=w741) -> ("Meas 2"=w737:dbl, "Meas 1"=w738:dbl)
          "kW" <- w738
          "?VkVAr" <- w737
          n493 = Bundle By Name(cluster=w735, "P3"=w738, "Q3"=w737) -> (w736:T4)
        }
        frame 1026 {
          w747 = 1000.0 ("factor 1")
          # "Q"
          # "P"
          n494 = call "U8arrayToMeasurement.vi"("factor 2"=w747, "factor 1"=w747, "payload"=w748) -> ("Meas 2"=w744:dbl, "Meas 1"=w745:dbl)
          "kW" <- w745
          "?VkVAr" <- w744
          n495 = Bundle By Name(cluster=w742, "P4"=w745, "Q4"=w744) -> (w743:T4)
        }
        frame 262 {
          w754 = 1.0 ("factor 1")
          n496 = call "U8arrayToMeasurement.vi"("factor 2"=w754, "factor 1"=w754, "payload"=w753) -> ("Meas 1"=w752:dbl)  [unwired: 1 out]
          n497 = Bundle By Name(cluster=w749, "Vdc1"=w752) -> (w750:T4)
        }
        frame 518 {
          w762 = 1.0 ("factor 1")
          # "Vdc"
          n498 = call "U8arrayToMeasurement.vi"("factor 2"=w762, "factor 1"=w762, "payload"=w761) -> ("Meas 2"=w759:dbl, "Meas 1"=w760:dbl)
          n499 = Add(x=w760, y=w759) -> (x+y=w758:dbl)
          n500 = Bundle By Name(cluster=w756, "Vdc2"=w758) -> (w755:T4)
        }
        frame 774 {
          w770 = 1.0 ("factor 1")
          # "Vdc"
          n501 = call "U8arrayToMeasurement.vi"("factor 2"=w770, "factor 1"=w770, "payload"=w769) -> ("Meas 2"=w767:dbl, "Meas 1"=w768:dbl)
          n502 = Add(x=w768, y=w767) -> (x+y=w763:dbl)
          n503 = Bundle By Name(cluster=w765, "Vdc3"=w763) -> (w764:T4)
        }
        frame 1030 {
          w778 = 1.0 ("factor 1")
          # "Vdc"
          n504 = call "U8arrayToMeasurement.vi"("factor 2"=w778, "factor 1"=w778, "payload"=w777) -> ("Meas 2"=w775:dbl, "Meas 1"=w776:dbl)
          n505 = Add(x=w776, y=w775) -> (x+y=w771:dbl)
          n506 = Bundle By Name(cluster=w772, "Vdc4"=w771) -> (w773:T4)
        }
      }
      n507 = local write "measurements"(w603) -> ()
      n508 = local write "conv"(w605) -> ()
      "CAN IN" <- w607
    }
    n509 = local read "main stop"() -> (w599:bool)
    n510 = node-c288() -> ()  [unwired: 1 in, 1 out]
  }
  n511 = call <instrlib>:"niSync Close.vi"("error in (no error)"=w20, "instrument handle"=w21) -> ("error out"=→"Error out":errorcluster)  [unwired: 9 in]
  n512 = UDP Close(connection ID=w1, 8:w6) -> ()  [unwired: 2 out]
  n513 = while {
    stop <- w781 stop-if-true
    n514 = flat-sequence {
      tunnel: [w783] -> w782
      tunnel: w782 -> [w790]
      frame #0 {
        n515 = local read "start following 1 pre"() -> (w784:bool)
        n516 = call <userlib>:"Boolean Trigger__ogtk.vi"("Boolean Input"=w784) -> ("Rising Edge"=w785:bool)  [unwired: 1 in, 1 out]
        n517 = case shown="True" w785 {
          tunnel: w784 -> [w786 w787]
          tunnel: [w786 w787] -> w783
          frame False {
          }
          frame True {
            n518 = Get Date/Time In Seconds() -> (seconds since 1Jan1904=→"time_afe":timestamp)
            n519 = Wait (ms)(milliseconds to wait=u32 550) -> ()  [unwired: 1 out]
          }
        }
      }
      frame #1 {
        n520 = local write "Start following 1"(w790) -> ()
      }
    }
    n521 = local read "main stop"() -> (w781:bool)
  }
  n522 = node-c288(w42) -> ()  [unwired: 1 out]
  n523 = node-c288(w37) -> ()  [unwired: 1 out]
  n524 = call <vilib>:"XNET Stop.vi"("session in"=w47) -> ()  [unwired: 13 in, 2 out]
  n525 = local write "CAN with Conv"(w45) -> ()
  n526 = call <vilib>:"XNET Stop.vi"("session in"=w48) -> ()  [unwired: 13 in, 2 out]
  n527 = UDP Close(connection ID=w10, 8:w9) -> ()  [unwired: 2 out]
  "Measurements" <- w34
  "CAN with Conv" <- w34
  "logging" <- w34
  "Ready 1" <- w34
  "OFF 1" <- w34
  "Ready 2" <- w34
  "ON 2" <- w34
  "OFF 2" <- w34
  "Ready 4" <- w34
  "ON 4" <- w34
  "OFF 4" <- w34
  "ON 3" <- w34
  "Ready 3" <- w34
  "OFF 3" <- w34
  "Fault 1" <- w34
  "Error 1" <- w34
  "Fault 2" <- w34
  "Error 2" <- w34
  "Fault 3" <- w34
  "Error 3" <- w34
  "Fault 4" <- w34
  "Error 4" <- w34
  "Forming 2" <- w28
  "Forming 1" <- w28
